vi "DSP_GetStatusFlags.vi"(0 "Board Handle":u64, 1 "error in (no error)":errorcluster) -> (2 "Board Handle Out":u64, 3 "FIFO from FFT overflow":bool, 4 "FIFO to FFT overflow":bool, 5 "error out":errorcluster)   [LabVIEW 2009]
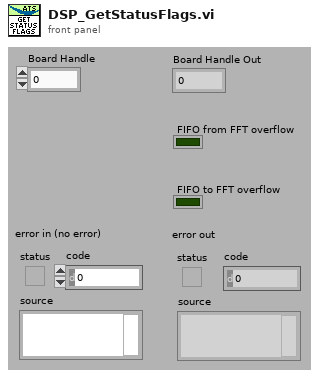
[diagram p1: front panel]
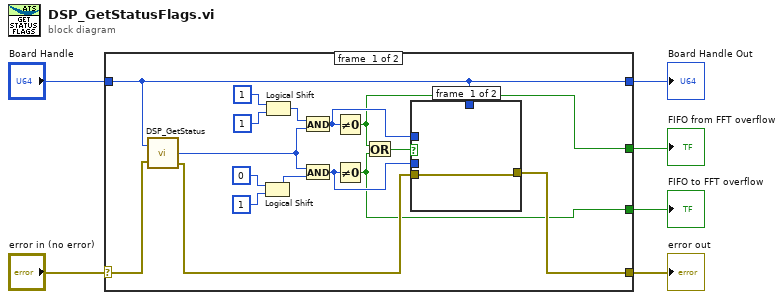
[diagram p0: block diagram]
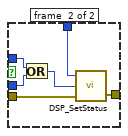
[diagram p2: hidden frame]
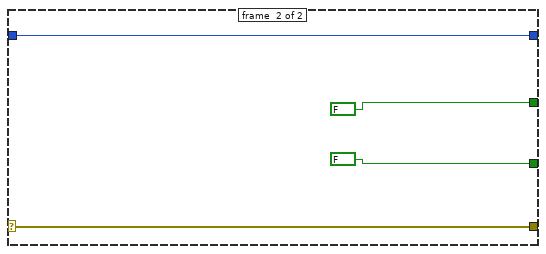
[diagram p3: hidden frame]
diagram:
  n1 = case shown="No Error" "error in (no error)" {
    selector: "error in (no error)" -> [w18 w33]
    tunnel: [w12 w33] -> w5
    tunnel: [w11 w32] -> w4
    tunnel: "Board Handle" -> [w11 w32]
    tunnel: [w7 FALSE] -> w2
    tunnel: [w8 FALSE] -> w1
    frame #0 {
      n2 = call "DSP_GetStatus.vi"("Board Handle"=w11, "error in (no error)"=w18) -> ("Status"=w15:u32, "error out"=w13:errorcluster)  [unwired: 1 out]
      n3 = Logical Shift(y=u32 0, x=u32 1) -> (x << y=w16:u32)
      n4 = Logical Shift(y=u32 1, x=u32 1) -> (x << y=w17:u32)
      n5 = And(x=w17, y=w15) -> (x .and. y?=w10:u32)
      n6 = And(x=w15, y=w16) -> (x .and. y?=w9:u32)
      n7 = Not Equal To 0?(x=w10) -> (x != 0?=w7:bool)
      n8 = Not Equal To 0?(x=w9) -> (x != 0?=w8:bool)
      n9 = Or(x=w7, y=w8) -> (x .or. y?=w14:bool)
      n10 = case shown="True" w14 {
        tunnel: w13 -> [w23 w29]
        tunnel: [w23 w28] -> w12
        tunnel: w11 -> [_ w27]
        tunnel: w10 -> [_ w26]
        tunnel: w9 -> [_ w25]
        frame #0 {
        }
        frame #1 {
          n11 = Or(x=w26, y=w25) -> (x .or. y?=w24:u32)
          n12 = call "DSP_SetStatus.vi"("error in (no error)"=w29, "Status"=w24, "Board Handle"=w27) -> ("error out"=w28:errorcluster)  [unwired: 1 out]
        }
      }
    }
    frame #1 {
    }
  }
  "Board Handle Out" <- w4
  "error out" <- w5
  "FIFO to FFT overflow" <- w1
  "FIFO from FFT overflow" <- w2
